vi "Reversing_an_array.vi"() -> ()   [LabVIEW 2019]
doc: "A vi that is used to reverse an array of random numbers without using the Revers 1D Array Function"
panel:
  out "Reversed Array":dbl[](array[numeric])
  in  "Array Size":i32=1
  out "Array of Random Numbers":dbl[](array[numeric])
  # "REVERSING AN ARRAY"
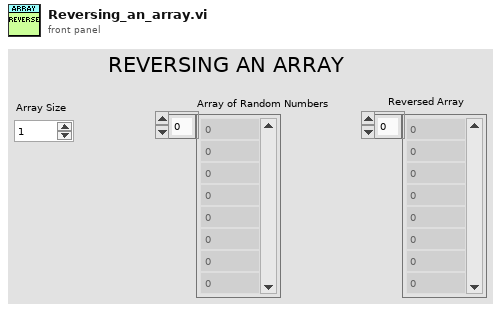
[diagram p1: front panel]
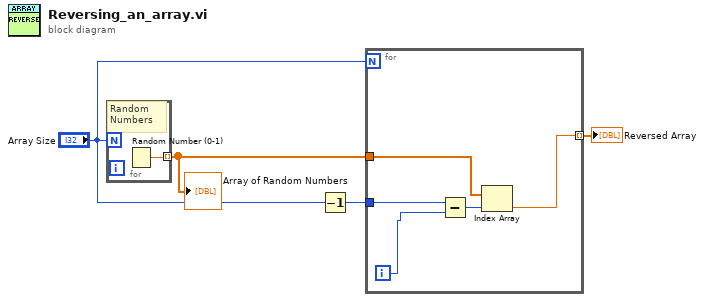
[diagram p0: block diagram]
diagram:
  n1 = for {
    N: "Array Size" -> [_]
    tunnel: [w5] -> w1 mode=indexing
    # "Random\nNumbers"
    n2 = Random Number (0-1)() -> (number: 0 to 1=w5:dbl)
  }
  "Array of Random Numbers" <- w1
  n3 = Decrement(x="Array Size") -> (x-1=w3:i32)
  n4 = for {
    N: "Array Size" -> [_]
    tunnel: w1 -> [w10]
    tunnel: w3 -> [w7]
    tunnel: [w6] -> w2 mode=indexing
    i -> [w8]
    n5 = Subtract(x=w7, y=w8) -> (x-y=w9:i32)
    n6 = Index Array(array=w10, index=w9) -> (element=w6:dbl)
  }
  "Reversed Array" <- w2
